vi "Class_Tree Tag_Encode.vi"(7 "Action":T2(ring)=enum."Terminal Properties", 8 "Property Type":T1(ring), 9 "Index":u16, 10 "Hierarchy":string, 11 "Unique ID string":string) -> (0 "Parents":string[](array[string]), 1 "Indent":i32, 2 "Tag":string, 3 "Display name":string)   [LabVIEW 2023]
doc: "By using the long name localized for the tag, children of search matches will be shown. ID is required in tag bc we set the property node terminals by ID.\n\nThe display valule will be the short name for property and method dialogs, and the full name for remove and rearrange dialongs.\n\nFormat is\n\nindex.propertyType.parent:shortName where parent:shortName=Long name (localized)\n\nAll properties classses and methods have a property item which contains the class/property heirarchy in a colon delimited list. This is used in sorting and filtering of items."
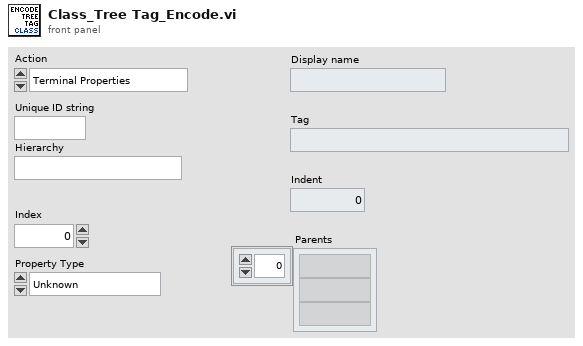
[diagram p1: front panel]
types:
  T1 = enum16{"Unknown", "Base", "Scripting", "Private", "Deprecated"}
  T2 = enum16{"[NONE]", "Wire Bundle", "Wire Unbundle", "Terminal Unbundle", "Terminal Bundle", "Bundler Insert", "Bundler Remove", "Bundler Rearrange", "In Place Insert", "In Place Remove", "In Place Rearrange", "Wire Properties", "Wire Method", "Terminal Properties", "Terminal Method", "Properties Insert", "Properties Remove", "Properties Rearrange", "Method Change", "Classes"}
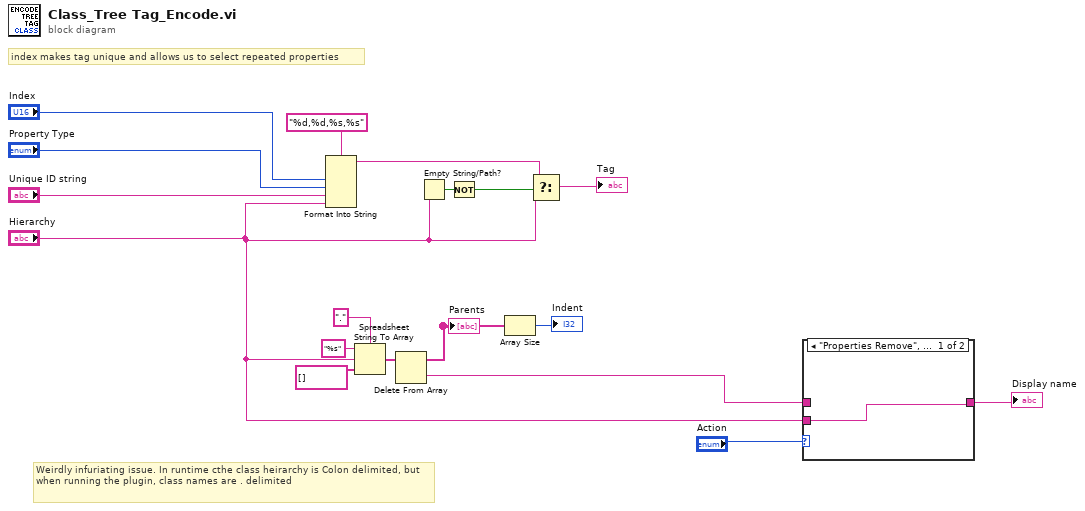
[diagram p0: block diagram]
diagram:
  # "Weirdly infuriating issue. In runtime cthe class heirarchy is Colon delimited, but when running the plugin, class names are . delimited"
  # "index makes tag unique and allows us to select repeated properties"
  n1 = Format Into String(format string="%d,%d,%s,%s", "Index", "Property Type", "Unique ID string", "Hierarchy") -> (resulting string=w17:string)  [unwired: 2 in, 1 out]
  n2 = Spreadsheet String To Array(delimiter (Tab)=".", format string="%s", spreadsheet string="Hierarchy", array type (2D Dbl)=string[] []) -> (array=w7:string[])
  n3 = Delete From Array(array=w7) -> (deleted portion=w3:string, array with subset deleted=w6:string[])  [unwired: 2 in]
  "Parents" <- w6
  n4 = Empty String/Path?(string/path="Hierarchy") -> (empty?=w15:bool)
  n5 = Not(x=w15) -> (.not. x?=w14:bool)
  n6 = Array Size(array=w6) -> (size(s)=→"Indent":i32)
  n7 = Select(t=w17, s=w14, f="Hierarchy") -> (s? t:f=→"Tag":string)
  n8 = case shown="\"Properties Remove\", \"Properties Rearrange\"" "Action" {
    tunnel: [w19 w20] -> w4
    tunnel: w3 -> [_ w20]
    tunnel: "Hierarchy" -> [w19 _]
    frame "Properties Remove", "Properties Rearrange" {
    }
    frame Default {
    }
  }
  "Display name" <- w4
